vi "vision state fg.vi"(2 "State In":T2, 3 "Menu":T1) -> (0 "State Out":T2, 1 "Enabled?":bool)   [LabVIEW 2014]
uses:
  typedefs/vision/vision enable.ctl
  typedefs/fg_getset.ctl
  vision.vi
panel:
  # "Interact With Vision Enable State Global Variable"
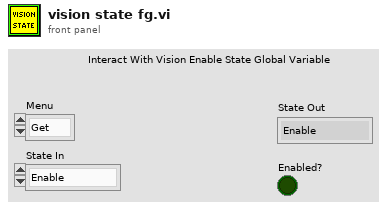
[diagram p1: front panel]
types:
  T1 = typedef "fg_getset.ctl" = enum16{"Get", "Set"}
  T2 = typedef "vision enable.ctl" = enum16{"Enable", "Disable", "Stop"}
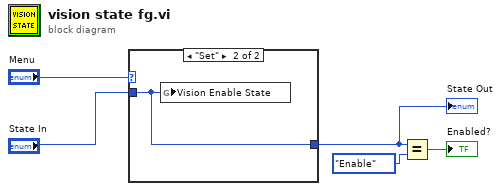
[diagram p0: block diagram]
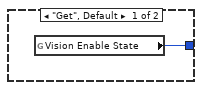
[diagram p2: hidden frame]
diagram:
  n1 = case shown="\"Set\"" "Menu" {
    tunnel: "State In" -> [_ w7]
    tunnel: [w6 w7] -> w1
    frame "Get", Default {
      n2 = global read "vision.vi" "Vision Enable State"() -> (w6:T2)
    }
    frame "Set" {
      n3 = global write "vision.vi" "Vision Enable State"(w7) -> ()
    }
  }
  "State Out" <- w1
  n4 = Equal?(x=w1, y=vision_enable."Enable") -> (x = y?=→"Enabled?":bool)
